vi "Drive_Set.vi"   [LabVIEW 2019]
uses:
  Globals/Drive_Globals.vi
  Drive_States.ctl
types:
  T1 = typedef "Drive_States.ctl" = enum16{"Percent_Voltage_Control", "Speed_Control"}
  T2 = typedef "Drive_Cluster.ctl" = cluster{"Control_State":T1, "Angular_Throttle":dbl, "Linear_Throttle":dbl, "Torque_Changing":bool}
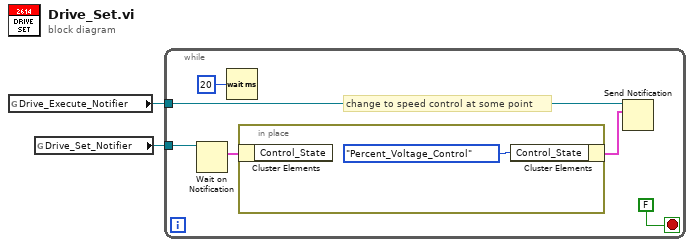
[diagram p0: block diagram]
diagram:
  n1 = global read "Drive_Globals.vi" "Drive_Execute_Notifier"() -> (w1:refnum<notifier>)
  n2 = global read "Drive_Globals.vi" "Drive_Set_Notifier"() -> (w2:refnum<notifier>)
  n3 = while {
    tunnel: w2 -> [w7]
    tunnel: w1 -> [w5]
    stop <- FALSE stop-if-true
    # "change to speed control at some point"
    n4 = Wait on Notification(notifier=w7) -> (notification=w6:T2)  [unwired: 3 in, 3 out]
    n5 = Wait (ms)(milliseconds to wait=u32 20) -> ()  [unwired: 1 out]
    n6 = in-place {
      n7 = in-place-cluster #1(w6) -> ()  [unwired: 1 out]
      n8 = in-place-cluster #1("Control_State"=Drive_States."Percent_Voltage_Control") -> (w4:T2)
    }
    n9 = Send Notification(notification=w4, notifier=w5) -> ()  [unwired: 1 in, 2 out]
  }
